vi "Read Symbolic Link.vi"(6 "timeout (ms)":i32=30000, 8 "error in":errorcluster, 10 "remote path":string, 11 "session in":refnum<class "Session.lvclass">) -> (0 "error out":errorcluster, 2 "remote target":string, 3 "session out":refnum<class "Session.lvclass">)   [LabVIEW 2020, in "NI_SFTP.lvlib"]
doc: "Resolves all symbolic links referenced in a remote path."
uses:
  <vilib>/net/SFTP/NI_SFTP.lvlib
  <vilib>/net/SFTP/Session/Session.lvclass
  <vilib>/Utility/Deadline/NI_Deadline.lvlib
  <vilib>/net/SFTP/API/Support/Command/SSH_FXP_READLINK/SSH_FXP_READLINK.lvclass
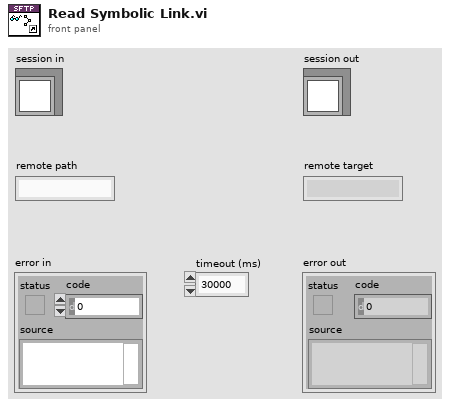
[diagram p1: front panel]
types:
  T1 = typedef "NI_Deadline.lvlib/Deadline.ctl" = cluster{"mode":T2, "deadline (ms)":u32}
  T2 = typedef "NI_Deadline.lvlib/Mode.ctl" = enum16{"Relative", "Use deadline", "Wait forever", "Nonblocking", "N/A"}
  T3 = typedef "NI_SFTP.lvlib/SSH_FXP_READLINK.lvclass/Output.ctl" = cluster{"file name":string, "long name":string}
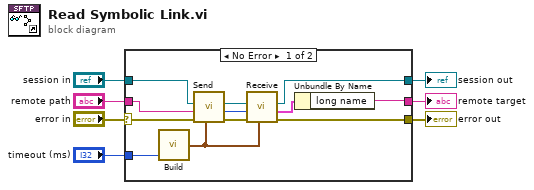
[diagram p0: block diagram]
diagram:
  n1 = case shown="No Error" "error in" {
    selector: "error in" -> [w19 w21]
    tunnel: [w15 w21] -> w5
    tunnel: [w10 w20] -> w1
    tunnel: "session in" -> [w12 w20]
    tunnel: "remote path" -> [w13 _]
    tunnel: "timeout (ms)" -> [w18 _]
    tunnel: [w8 _] -> w2
    frame No Error {
      n2 = call <vilib>:"Build.vi"("timeout (ms)"=w18) -> ("Deadline out"=w14:T1)  [unwired: 2 in]
      n3 = call <vilib>:"Send.vi"("Timeout"=w14, "error in (no error)"=w19, "path"=w13, "session in"=w12) -> ("error out"=w16:errorcluster, "request id"=w11:u32, "session out"=w17:refnum<class "Session.lvclass">)  [unwired: 4 in, 1 out]
      n4 = call <vilib>:"Receive.vi"("deadline"=w14, "error in (no error)"=w16, "request id"=w11, "session in"=w17) -> ("error out"=w15:errorcluster, "output"=w9:T3, "session out"=w10:refnum<class "Session.lvclass">)  [unwired: 4 in, 1 out]
      n5 = Unbundle By Name(w9) -> ("long name"=w8:string)
    }
    frame Error {
    }
  }
  "error out" <- w5
  "session out" <- w1
  "remote target" <- w2
